vi "Generate File Name.vi"(7 "file count":i32, 10 "name or relative path":string="Test.tif", 11 "base path":path=path "C:/Users/BoasLab/Documents/Data/Alazar data/B-line") -> (3 "appended path":path)   [LabVIEW 2018]
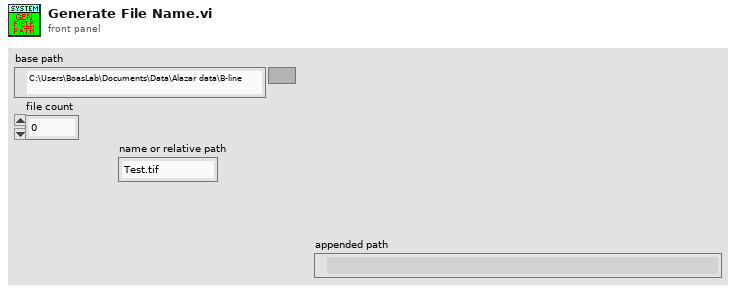
[diagram p1: front panel]
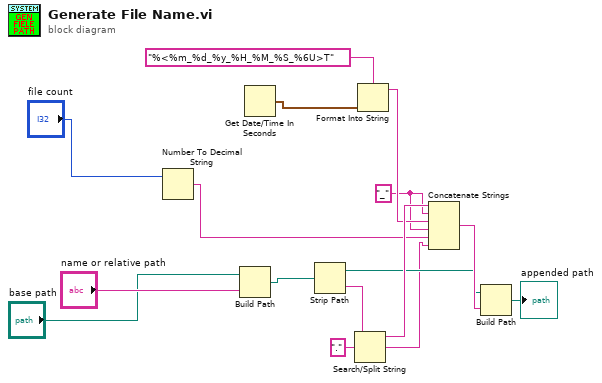
[diagram p0: block diagram]
diagram:
  w2 = "_" ("string")
  n1 = Number To Decimal String(number="file count") -> (decimal integer string=w1:string)  [unwired: 1 in]
  n2 = Build Path(base path="base path", name or relative path="name or relative path") -> (appended path=w9:path)
  n3 = Get Date/Time In Seconds() -> (seconds since 1Jan1904=w8:timestamp)
  n4 = Strip Path(path=w9) -> (stripped path=w12:path, name=w16:string)
  n5 = Search/Split String(string=w16, search string/char (-)=".") -> (substring before match=w14:string, match + rest of string=w3:string)  [unwired: 1 in, 1 out]
  n6 = Format Into String(format string="%<%m_%d_%y_%H_%M_%S_%6U>T", w8) -> (resulting string=w6:string)  [unwired: 2 in, 1 out]
  n7 = Concatenate Strings(w14, w2, w6, w2, w1, w3) -> (w13:string)
  n8 = Build Path(base path=w12, name or relative path=w13) -> (appended path=→"appended path":path)
